vi "ReportTCPConnectionTimeout.vi"(8 "error in (no error)":errorcluster, 9 "wait before close (500 ms)":u32=500, 11 "connection ID":refnum<k5>) -> (0 "error out":errorcluster, 3 "connection ID out":refnum<k5>)   [LabVIEW 2013]
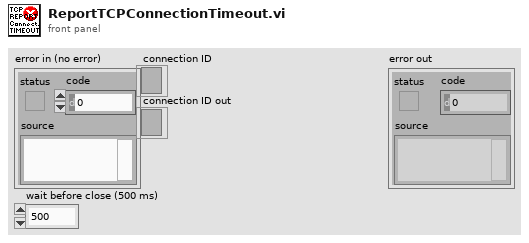
[diagram p1: front panel]
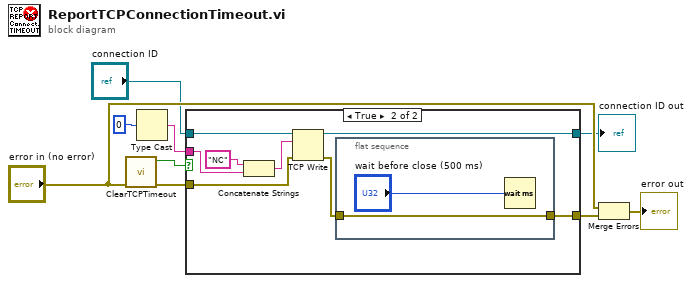
[diagram p0: block diagram]
diagram:
  n1 = call "ClearTCPTimeout.vi"("error in (no error)"="error in (no error)") -> ("error out"=w8:errorcluster, "TCP Timeout?"=w9:bool)  [unwired: 9 in]
  n2 = Type Cast(x=0) -> (*(type *) &x=w2:string)  [unwired: 1 in]
  n3 = case shown="True" w9 {
    tunnel: w8 -> [w11 w17]
    tunnel: [w11 w13] -> w6
    tunnel: "connection ID" -> [w10 w16]
    tunnel: [w10 w12] -> w4
    tunnel: w2 -> [_ w18]
    frame False {
    }
    frame True {
      n4 = Concatenate Strings("NC" ("string"), w18) -> (w15:string)
      n5 = TCP Write(connection ID=w16, data in=w15, error in (no error)=w17) -> (connection ID out=w12:refnum<k5>, error out=w14:errorcluster)  [unwired: 1 in, 1 out]
      n6 = flat-sequence {
        tunnel: w14 -> [w21]
        tunnel: [w21] -> w13
        frame #0 {
          n7 = Wait (ms)(milliseconds to wait="wait before close (500 ms)") -> ()  [unwired: 1 out]
        }
      }
    }
  }
  "connection ID out" <- w4
  n8 = Merge Errors("error in (no error)", w6) -> (→"error out":errorcluster)
